vi "PH_Beckhoff_PP_PU.set Hardware reconfigured.vi"(0 "i ref in":refnum<vi>, 2 "Hardware reconfigured?":bool, 5 "error in":errorcluster) -> (14 "i ref out":refnum<vi>, 19 "error out":errorcluster)   [LabVIEW 2014, in "PH_Beckhoff_PP_PU.lvlib"]
doc: "This VI writes information to own attributes and sets the related GUI elements."
uses:
  PH_Beckhoff_PP_PU.lvlib
  PH_Basics/PH_Common/PH_Common.lvlib
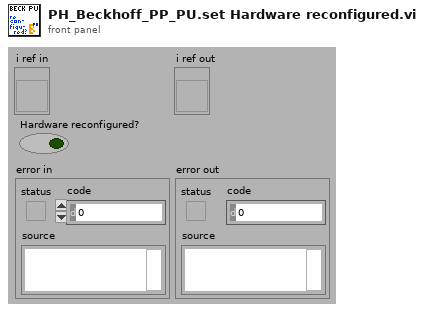
[diagram p1: front panel]
types:
  T1 = typedef "PH_Beckhoff_PP_PU.lvlib/PH_Beckhoff_PP_PU.i attribute.ctl" = cluster{"HV Meas":cluster{"Input GUI Ref":refnum<vi>, "Voltage Service ID":i32, "Voltage [V]":dbl, "Quality":bool, "# in Data":i32}[], "Trigger":cluster{"Status":cluster{"GUI Ref":refnum<vi>, "Status Service ID":i32, "Status":T2}, "last shot:":cluster{"GUI Ref":refnum<vi>, "Service ID":i32, "Time":string}, "DIs":cluster{"triggered":cluster{"GUI Ref":refnum<vi>, "# in Data":i32}, "fired":cluster{"GUI Ref":refnum<vi>, "# in Data":i32}}, "GUI Ref Indicator":refnum<vi>}[], "RR":cluster{"Status":cluster{"GUI Ref":refnum<vi>, "Status Service ID":i32, "Status":T2}, "DIs":cluster{"closed":cluster{"GUI Ref":refnum<vi>, "# in Data":i32}, "open":cluster{"GUI Ref":refnum<vi>, "# in Data":i32}}, "Close":cluster{"GUI Ref":refnum<vi>, "# in Data":i32}, "GUI Ref Indicator":refnum<vi>}[], "Igni":cluster{"Status":cluster{"GUI Ref":refnum<vi>, "Status Service ID":i32, "Status":T2}, "DIs":cluster{"heating on":cluster{"GUI Ref":refnum<vi>, "# in Data":i32}, "water on":cluster{"GUI Ref":refnum<vi>, "# in Data":i32}}, "Device on":cluster{"GUI Ref":refnum<vi>, "# in Data":i32}, "GUI Ref Indicator":refnum<vi>}[], "PSU":cluster{"Status":cluster{"GUI Ref":refnum<vi>, "Status Service ID":i32, "Status":T2}, "Limit Service ID":i32, "DIs":cluster{"inhibit":cluster{"GUI Ref":refnum<vi>, "# in Data":i32}, "end of charge":cluster{"GUI Ref":refnum<vi>, "# in Data":i32}, "HV on":cluster{"GUI Ref":refnum<vi>, "# in Data":i32}, "overtemp":cluster{"GUI Ref":refnum<vi>, "# in Data":i32}, "interlock":cluster{"GUI Ref":refnum<vi>, "# in Data":i32}, "load fault":cluster{"GUI Ref":refnum<vi>, "# in Data":i32}, "sum fault":cluster{"GUI Ref":refnum<vi>, "# in Data":i32}, "HV off":cluster{"GUI Ref":refnum<vi>, "# in Data":i32}, "DC ok":cluster{"GUI Ref":refnum<vi>, "# in Data":i32}}, "AIs":cluster{"voltage":cluster{"GUI Ref":refnum<vi>, "# in Data":i32}, "current":cluster{"GUI Ref":refnum<vi>, "# in Data":i32}}, "DAs":cluster{"inhibit":cluster{"GUI Ref":refnum<vi>, "# in Data":i32}, "interlock":cluster{"GUI Ref":refnum<vi>, "# in Data":i32}, "HV on":cluster{"GUI Ref":refnum<vi>, "# in Data":i32}, "Reset":cluster{"GUI Ref":refnum<vi>, "# in Data":i32}}, "AAs":cluster{"Voltage to set":cluster{"GUI Ref":refnum<vi>, "# in Data":i32}}, "GUI Ref Indicator":refnum<vi>}[], "reconfigured":cluster{"?":bool, "GUI Ref":refnum<vi>}, "PU Rack Type":T3, "HV Meas Info":T4, "PSU Info":T5}
  T2 = typedef "PH_StatusHandler.lvlib/PH_StatusHandler.Status.ctl" = i16
  T3 = typedef "PH_Beckhoff_PP_PU.lvlib/PH_Beckhoff_PP_PU.PU Rack Type.ctl" = enum16{"no Info", "PA 19mm", "PA 45mm", "MA PU 1 and 2", "MA PU 3 and 4", "MA PU 5 and 6", "MA FR and PILC"}
  T4 = typedef "PH_Beckhoff_PP_PU.lvlib/PH_Beckhoff_PP_PU.HV Meas Info.ctl" = cluster{"Period Time [s]":dbl, "Subtractor 1 [Hz]":dbl, "Devider 1 [Hz/kV]":dbl, "Subtractor 2 [Hz]":dbl, "Devider 2 [Hz/kV]":dbl}
  T5 = typedef "PH_Beckhoff_PP_PU.lvlib/PH_Beckhoff_PP_PU.PSU Info.ctl" = cluster{"Limits 1 [V]":cluster{"Lower":dbl, "Upper":dbl}, "Limits 2 [V]":cluster{"Lower":dbl, "Upper":dbl}}
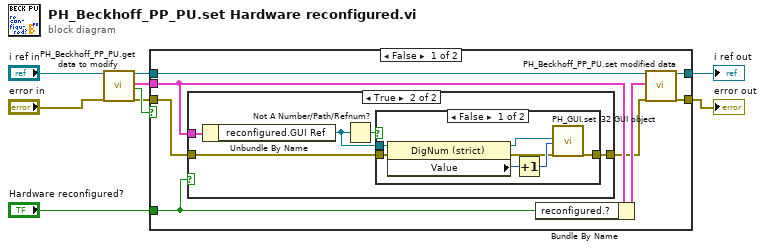
[diagram p0: block diagram]
diagram:
  n1 = call "PH_Beckhoff_PP_PU.get data to modify.vi"("i ref in"="i ref in", "error in (no error)"="error in") -> ("i ref out"=w3:refnum<vi>, "i attribute"=w8:T1, "timed out"=w7:bool, "error out"=w4:errorcluster)  [unwired: 14 in]
  n2 = case shown="False" w7 {
    tunnel: w3 -> [w17 w33]
    tunnel: w4 -> [w14 w32]
    tunnel: [w16 w33] -> w2
    tunnel: [w15 w32] -> w1
    tunnel: w8 -> [w13 _]
    tunnel: "Hardware reconfigured?" -> [w10 _]
    frame False {
      n3 = case shown="True" w10 {
        tunnel: w14 -> [w18 w23]
        tunnel: w13 -> [_ w22]
        tunnel: [w18 w19] -> w11
        frame False {
        }
        frame True {
          n4 = Unbundle By Name(w22) -> ("reconfigured.GUI Ref"=w21:refnum<vi>)
          n5 = Not A Number/Path/Refnum?(number/path/refnum=w21) -> (NaN/Path/Refnum?=w20:bool)
          n6 = case shown="False" w20 {
            tunnel: w23 -> [w30 w31]
            tunnel: [w25 w31] -> w19
            tunnel: w21 -> [w29 _]
            frame False {
              n7 = property class="DigNum (strict)"(reference=w29, error in=w30) -> (reference out=w24:refnum<vi>, error out=w26:errorcluster, "Value"=w28:i32)
              n8 = Increment(x=w28) -> (x+1=w27:i32)
              n9 = call "PH_GUI.set I32 GUI object.vi"("I32 GUI Ref"=w24, "value"=w27, "error in (no error)"=w26) -> ("error out"=w25:errorcluster)  [unwired: 16 in]
            }
            frame True {
            }
          }
        }
      }
      n10 = Bundle By Name(cluster=w13, "reconfigured.?"=w10) -> (w12:T1)
      n11 = call "PH_Beckhoff_PP_PU.set modified data.vi"("i ref in"=w17, "i attribute"=w12, "error in (no error)"=w11) -> ("i ref out"=w16:refnum<vi>, "error out"=w15:errorcluster)  [unwired: 15 in]
    }
    frame True {
    }
  }
  "i ref out" <- w2
  "error out" <- w1
